vi "80 Switch Input.vi"() -> ()   [LabVIEW 2018]
uses:
  <vilib>/Rock Robotics/WPI/Joystick/WPI_JoystickDeviceEnum.ctl
  <vilib>/Rock Robotics/SystemInterfaces/DIO/FPGA_DIOPWMChannel.ctl
  <vilib>/Rock Robotics/SystemInterfaces/DIO/FPGA_DIOChannel.ctl
  <vilib>/Rock Robotics/WPI/MotorControl/WPI_MotorControlOpen Talon.vi
  <vilib>/Rock Robotics/WPI/Switch/WPI_SwitchOpenLimit.vi
  <vilib>/Rock Robotics/WPI/MotorControl/WPI_MotorControlOpen SPARK.vi
panel:
  in  "Wrist Out Speed":dbl=0.5
  in  "Wrist In Speed":dbl=0.5
  out "POVs":i16[](array[numeric])
  out "Buttons":bool[](array[boolean])
  out "Axes":dbl[](array[numeric])
  in  "stop":bool
  out "Output":dbl(slide) scale=0.0..1.0
  out "Joystick X":dbl(slide) scale=1.0..-1.0
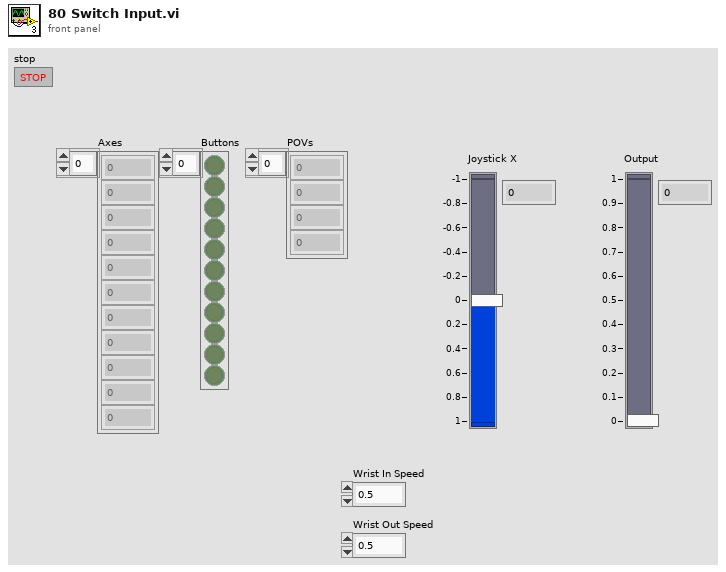
[diagram p1: front panel]
types:
  T1 = typedef "FPGA_DIOPWMChannel.ctl" = enum8{"PWM 0", "PWM 1", "PWM 2", "PWM 3", "PWM 4", "PWM 5", "PWM 6", "PWM 7", "PWM 8", "PWM 9", "PWM MXP 0", "PWM MXP 1", "PWM MXP 2", "PWM MXP 3", "PWM MXP 4", "PWM MXP 5", "PWM MXP 6", "PWM MXP 7", "PWM MXP 8", "PWM MXP 9", "Invalid"}
  T2 = typedef "FPGA_DIOChannel.ctl" = enum8{"DIO 0", "DIO 1", "DIO 2", "DIO 3", "DIO 4", "DIO 5", "DIO 6", "DIO 7", "DIO 8", "DIO 9", "DIO MXP 0", "DIO MXP 1", "DIO MXP 2", "DIO MXP 3", "DIO MXP 4", "DIO MXP 5", "DIO MXP 6", "DIO MXP 7", "DIO MXP 8", "DIO MXP 9", "DIO MXP 10", "DIO MXP 11", "DIO MXP 12", "DIO MXP 13", "DIO MXP 14", "DIO MXP 15", "SPI Port CS1", "SPI Port CS2", "SPI Port CS3", "SPI Port MISO", "SPI Port MOSI", "Invalid"}
  T3 = typedef "WPI_JoystickDeviceEnum.ctl" = enum16{"USB 0", "USB 1", "USB 2", "USB 3", "USB 4", "USB 5"}
  T4 = typedef "WPI_SwitchDevRef.ctl" = cluster{"DevStatus":errorcluster, "DIO Channel":T2, "CntIndex":T5, "Normally Closed":bool}
  T5 = typedef "FPGA_CounterCtrSystemIndex.ctl" = enum8{"Ctr 0", "Ctr 1", "Ctr 2", "Ctr 3", "Ctr 4", "Ctr 5", "Ctr 6", "Ctr 7", "Invalid"}
  T6 = typedef "WPI_MotorControlDeviceRef.ctl" = cluster{"DeviceStatus":errorcluster, "Type":T7, "PWM":cluster{"PWM Channel":T1, "DeadBand":T8}, "CAN":cluster{"Device Number":u8, "SetOutput VI Ref":variant, "GetOutput VI Ref":variant, "Enable VI Ref":variant, "Disable VI Ref":variant, "Data":variant}, "Invert":bool, "DIO PWM":cluster{"PWM \"Enable\" Channel":T1, "DIOChannel":T2, "PWM Rate":dbl}}
  T7 = typedef "WPI_MotorControlType.ctl" = enum16{"PWM", "CAN", "DIO PWM"}
  T8 = typedef "WPI_PWMDeadband.ctl" = cluster{"Name":string, "maxPositivePwm":i32, "minPositivePwm":i32, "centerPwm":i32, "maxNegativePwm":i32, "minNegativePwm":i32, "angularRange":u16}
  T9 = typedef "WPI_JoystickDevRef.ctl" = cluster{"Device":T3}
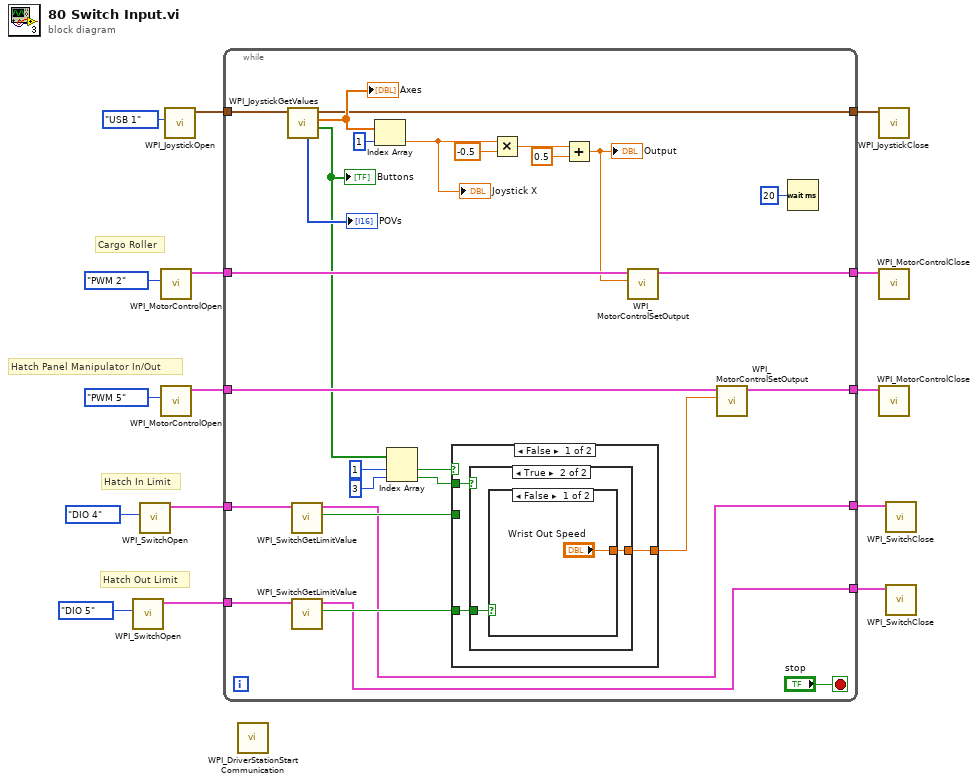
[diagram p0: block diagram]
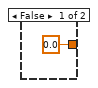
[diagram p2: hidden frame]
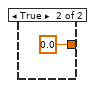
[diagram p3: hidden frame]
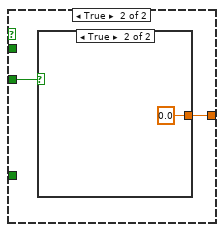
[diagram p4: hidden frame]
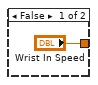
[diagram p5: hidden frame]
diagram:
  # "Hatch Panel Manipulator In/Out"
  # "Cargo Roller"
  # "Hatch Out Limit"
  # "Hatch In Limit"
  n1 = call-poly <vilib>:"WPI_SwitchOpen.vi"("DIO Channel"=FPGA_DIOChannel."DIO 5") -> ("SwitchDevRef"=w6:T4)  [unwired: 9 in, 1 out]
  n2 = call-poly <vilib>:"WPI_SwitchOpen.vi"("DIO Channel"=FPGA_DIOChannel."DIO 4") -> ("SwitchDevRef"=w7:T4)  [unwired: 9 in, 1 out]
  n3 = call-poly <vilib>:"WPI_MotorControlOpen.vi"("PWM Channel"=FPGA_DIOPWMChannel."PWM 2") -> ("MotorControlDeviceRef"=w11:T6)  [unwired: 9 in, 1 out]
  n4 = call-poly <vilib>:"WPI_MotorControlOpen.vi"("PWM Channel"=FPGA_DIOPWMChannel."PWM 5") -> ("MotorControlDeviceRef"=w4:T6)  [unwired: 9 in, 1 out]
  n5 = call <vilib>:"WPI_JoystickOpen.vi"("JoystickDevice"=WPI_JoystickDeviceEnum."USB 1") -> ("JoystickDevRef"=w14:T9)  [unwired: 10 in]
  n6 = while {
    tunnel: w14 -> [w38]
    tunnel: [w34] -> w13
    tunnel: w11 -> [w32]
    tunnel: [w30] -> w10
    tunnel: w7 -> [w29]
    tunnel: w6 -> [w28]
    tunnel: w4 -> [w26]
    tunnel: [w27] -> w5
    tunnel: [w17] -> w2
    tunnel: [w16] -> w1
    stop <- "stop" stop-if-true
    n7 = call <vilib>:"WPI_JoystickGetValues.vi"("JoystickDevRef"=w38) -> ("Buttons"=w25:bool[], "Axes"=w37:dbl[], "JoystickDevRef"=w34:T9, "POVs"=→"POVs":i16[])  [unwired: 6 in, 1 out]
    "Axes" <- w37
    "Buttons" <- w25
    n8 = call <vilib>:"WPI_SwitchGetLimitValue.vi"("SwitchDevRef"=w29) -> ("Switch Pressed"=w21:bool, "SwitchDevRef"=w17:T4)  [unwired: 8 in, 1 out]
    n9 = call <vilib>:"WPI_SwitchGetLimitValue.vi"("SwitchDevRef"=w28) -> ("Switch Pressed"=w18:bool, "SwitchDevRef"=w16:T4)  [unwired: 8 in, 1 out]
    n10 = Index Array(array=w37, index=1) -> (element=w35:dbl)
    "Joystick X" <- w35
    n11 = Index Array(array=w25, index #1=1 ("index"), index #2=3 ("index")) -> (element #1=w22:bool, element #2=w19:bool)
    n12 = case shown="False" w22 {
      tunnel: w21 -> [_ w53]
      tunnel: [w44 w52] -> w20
      tunnel: w19 -> [w46 _]
      tunnel: w18 -> [w45 _]
      frame False {
        n13 = case shown="True" w46 {
          tunnel: w45 -> [_ w49]
          tunnel: [0.0 ("Wrist Out Speed") w48] -> w44
          frame False {
          }
          frame True {
            n14 = case shown="False" w49 {
              tunnel: ["Wrist Out Speed" 0.0] -> w48
              frame False {
              }
              frame True {
              }
            }
          }
        }
      }
      frame True {
        n15 = case shown="True" w53 {
          tunnel: ["Wrist In Speed" 0.0] -> w52
          frame False {
          }
          frame True {
          }
        }
      }
    }
    n16 = Multiply(x=w35, y=-0.5) -> (x*y=w40:dbl)
    n17 = Add(x=w40, y=0.5) -> (x+y=w31:dbl)
    "Output" <- w31
    n18 = call <vilib>:"WPI_MotorControlSetOutput.vi"("Output"=w31, "MotorControlDevRef"=w32) -> ("MotorControlDevRef"=w30:T6)  [unwired: 7 in, 2 out]
    n19 = call <vilib>:"WPI_MotorControlSetOutput.vi"("Output"=w20, "MotorControlDevRef"=w26) -> ("MotorControlDevRef"=w27:T6)  [unwired: 7 in, 2 out]
    n20 = Wait (ms)(milliseconds to wait=u32 20) -> ()  [unwired: 1 out]
  }
  n21 = call <vilib>:"WPI_DriverStationStart Communication.vi"() -> ()  [unwired: 12 in]
  n22 = call <vilib>:"WPI_JoystickClose.vi"("JoystickDevRef"=w13) -> ()  [unwired: 11 in]
  n23 = call <vilib>:"WPI_MotorControlClose.vi"("MotorControlDevRef"=w10) -> ()  [unwired: 10 in, 1 out]
  n24 = call <vilib>:"WPI_MotorControlClose.vi"("MotorControlDevRef"=w5) -> ()  [unwired: 10 in, 1 out]
  n25 = call <vilib>:"WPI_SwitchClose.vi"("SwitchDevRef"=w2) -> ()  [unwired: 10 in, 1 out]
  n26 = call <vilib>:"WPI_SwitchClose.vi"("SwitchDevRef"=w1) -> ()  [unwired: 10 in, 1 out]
